vi "CLD Timer.vi"(8 "error in":errorcluster, 10 "Time Target (s)":dbl format="%#_13g", 11 "CLD 12 Timer Enum":T1) -> (0 "error out":errorcluster, 2 "Has Time Elapsed?":bool, 3 "Elapsed Time":dbl)   [LabVIEW 2018]
uses:
  CLD12 Timer Enum.ctl
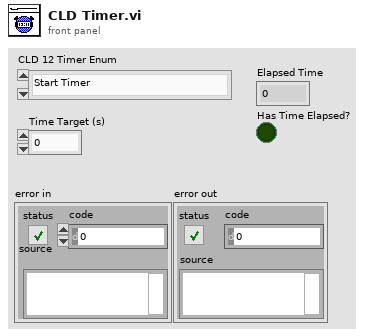
[diagram p1: front panel]
types:
  T1 = typedef "CLD12 Timer Enum.ctl" = enum16{"Start Timer", "Read Time", "Pause", "UnPause", "Reset Timer"}
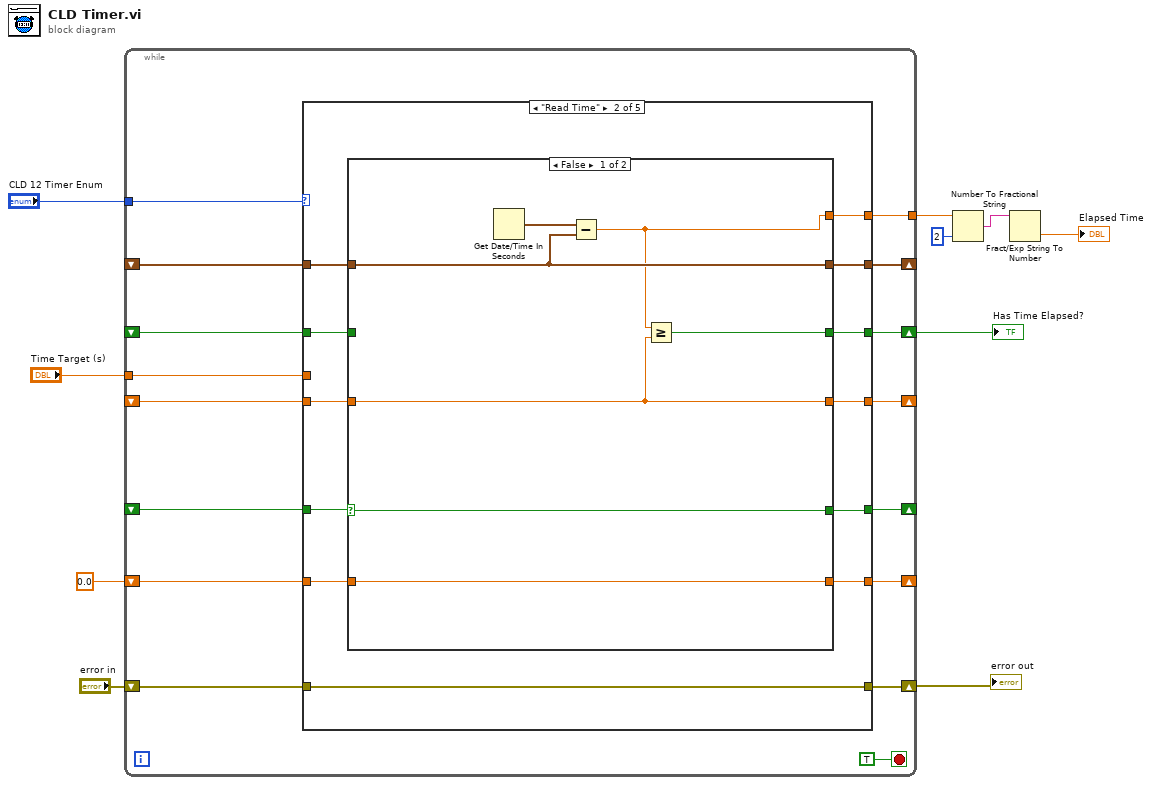
[diagram p0: block diagram]
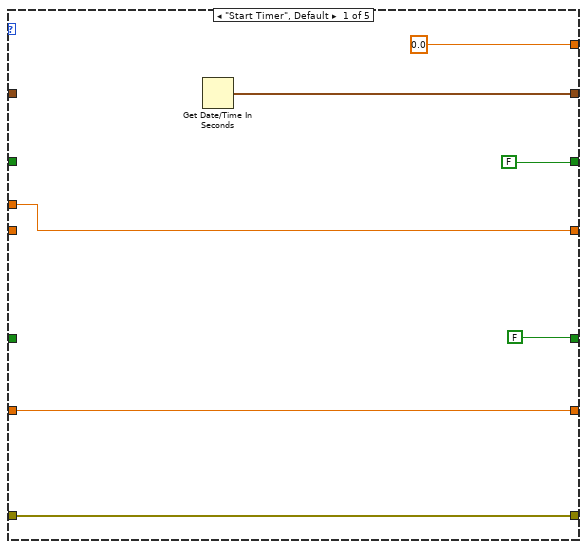
[diagram p2: hidden frame]
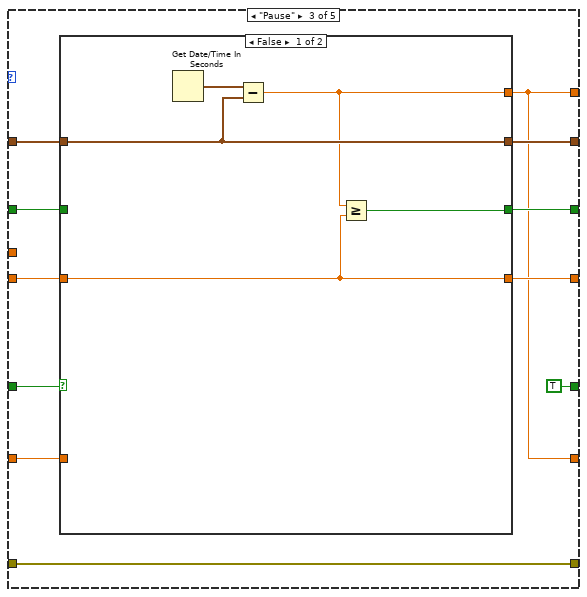
[diagram p4: hidden frame]
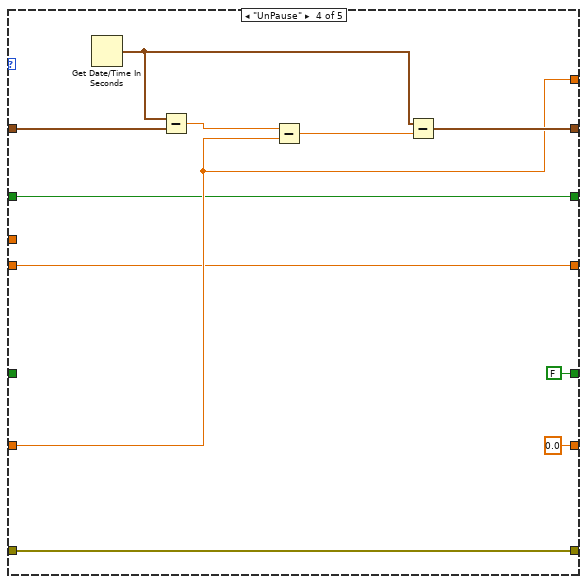
[diagram p6: hidden frame]
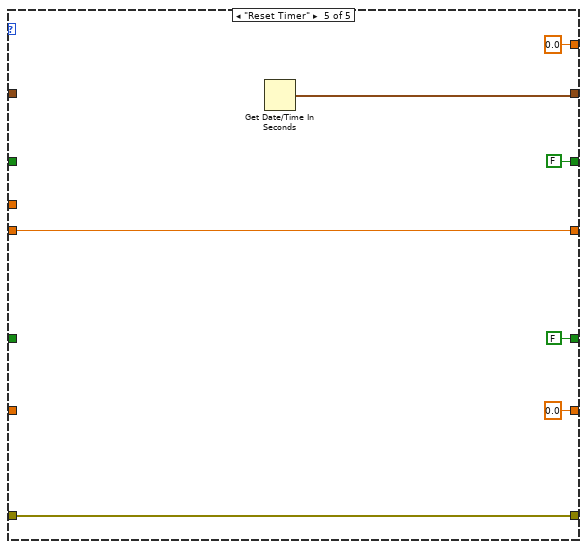
[diagram p7: hidden frame]
diagram:
  n1 = while {
    shift-right: [w25] -> w9
    shift-left: "error in" -> [w26]
    tunnel: "CLD 12 Timer Enum" -> [w24]
    shift-right: [w23] -> _
    shift-left: _ -> [w22]
    shift-right: [w20] -> w1
    shift-left: _ -> [w21]
    tunnel: "Time Target (s)" -> [w19]
    shift-right: [w17] -> _
    shift-left: _ -> [w18]
    shift-right: [w15] -> _
    shift-left: _ -> [w16]
    shift-right: [w13] -> _
    shift-left: 0.0 -> [w14]
    tunnel: [w11] -> w5
    stop <- TRUE stop-if-true
    n2 = case shown="\"Read Time\"" w24 {
      tunnel: w26 -> [w27 w45 w68 w78 w89]
      tunnel: [w27 w45 w68 w78 w89] -> w25
      tunnel: [w33 w42 w59 w84 w90] -> w23
      tunnel: w22 -> [_ w43 w60 w88 _]
      tunnel: w21 -> [_ w41 w62 w82 _]
      tunnel: [FALSE w40 w61 w82 FALSE] -> w20
      tunnel: w19 -> [w31 _ _ _ _]
      tunnel: w18 -> [_ w39 w64 w81 w91]
      tunnel: [w31 w38 w63 w81 w91] -> w17
      tunnel: w16 -> [_ w44 w67 _ _]
      tunnel: [FALSE w37 TRUE FALSE FALSE] -> w15
      tunnel: w14 -> [w29 w36 w66 w83 _]
      tunnel: [w29 w35 w58 0.0 0.0] -> w13
      tunnel: [0.0 w34 w58 w83 0.0] -> w11
      frame "Start Timer", Default {
        n3 = Get Date/Time In Seconds() -> (seconds since 1Jan1904=w33:timestamp)
      }
      frame "Read Time" {
        n4 = case shown="False" w44 {
          selector: w44 -> [w48 w54]
          tunnel: w43 -> [w51 w57]
          tunnel: [w51 w57] -> w42
          tunnel: w41 -> [_ w56]
          tunnel: [w49 w56] -> w40
          tunnel: w39 -> [w50 w55]
          tunnel: [w50 w55] -> w38
          tunnel: [w48 w54] -> w37
          tunnel: w36 -> [w47 w53]
          tunnel: [w47 w53] -> w35
          tunnel: [w46 w53] -> w34
          frame False {
            n5 = Get Date/Time In Seconds() -> (seconds since 1Jan1904=w52:timestamp)
            n6 = Subtract(x=w52, y=w51) -> (x-y=w46:dbl)
            n7 = Greater Or Equal?(x=w46, y=w50) -> (x >= y?=w49:bool)
          }
          frame True {
          }
        }
      }
      frame "Pause" {
        n8 = case shown="False" w67 {
          tunnel: w66 -> [_ w74]
          tunnel: [w69 w74] -> w58
          tunnel: w64 -> [w71 w77]
          tunnel: [w71 w77] -> w63
          tunnel: w62 -> [_ w76]
          tunnel: [w70 w76] -> w61
          tunnel: w60 -> [w72 w75]
          tunnel: [w72 w75] -> w59
          frame False {
            n9 = Get Date/Time In Seconds() -> (seconds since 1Jan1904=w73:timestamp)
            n10 = Subtract(x=w73, y=w72) -> (x-y=w69:dbl)
            n11 = Greater Or Equal?(x=w69, y=w71) -> (x >= y?=w70:bool)
          }
          frame True {
          }
        }
      }
      frame "UnPause" {
        n12 = Get Date/Time In Seconds() -> (seconds since 1Jan1904=w85:timestamp)
        n13 = Subtract(x=w85, y=w88) -> (x-y=w87:dbl)
        n14 = Subtract(x=w87, y=w83) -> (x-y=w86:dbl)
        n15 = Subtract(x=w85, y=w86) -> (x-y=w84:timestamp)
      }
      frame "Reset Timer" {
        n16 = Get Date/Time In Seconds() -> (seconds since 1Jan1904=w90:timestamp)
      }
    }
  }
  "error out" <- w9
  "Has Time Elapsed?" <- w1
  n17 = Number To Fractional String(number=w5, precision (6)=i16 2) -> (F-format string=w3:string)  [unwired: 2 in]
  n18 = Fract/Exp String To Number(string=w3) -> (number=→"Elapsed Time":dbl)  [unwired: 3 in, 1 out]
